vi "Recursive Add Item References to Map.vi"(8 "error in (no error)":errorcluster, 10 "ProjectItem Refnum":refnum<vi>, 11 "Icon Decorator In":refnum<class "Icon Decorator.lvclass">) -> (0 "error out":errorcluster, 3 "Icon Decorator Out":refnum<class "Icon Decorator.lvclass">)   [LabVIEW 2020, in "Icon Decorator.lvlib" / "Icon Decorator.lvclass"]
uses:
  Icon Decorator.lvclass
  Icon Decorator.lvclass/Icon Decorator.ctl
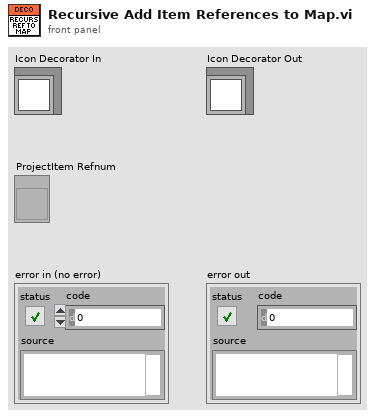
[diagram p1: front panel]
types:
  T1 = typedef "ItemRef.ctl" = u64
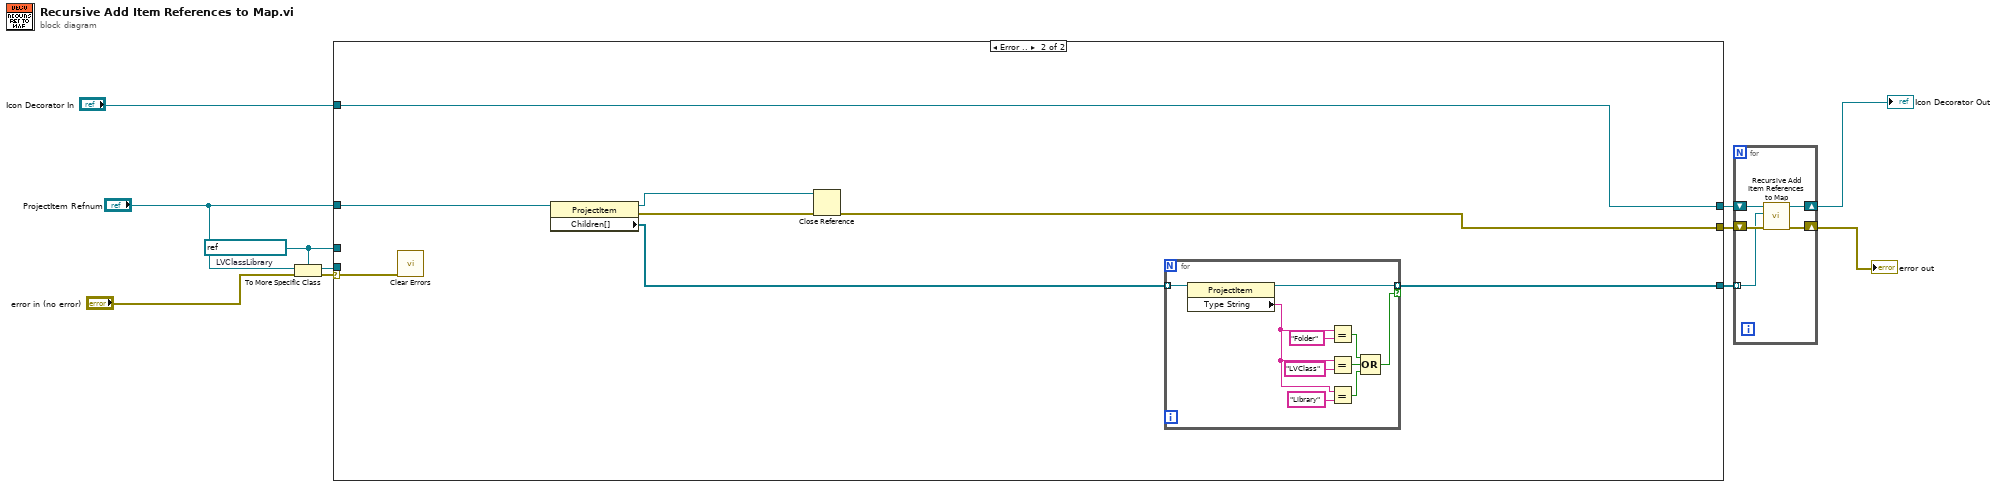
[diagram p0: block diagram]
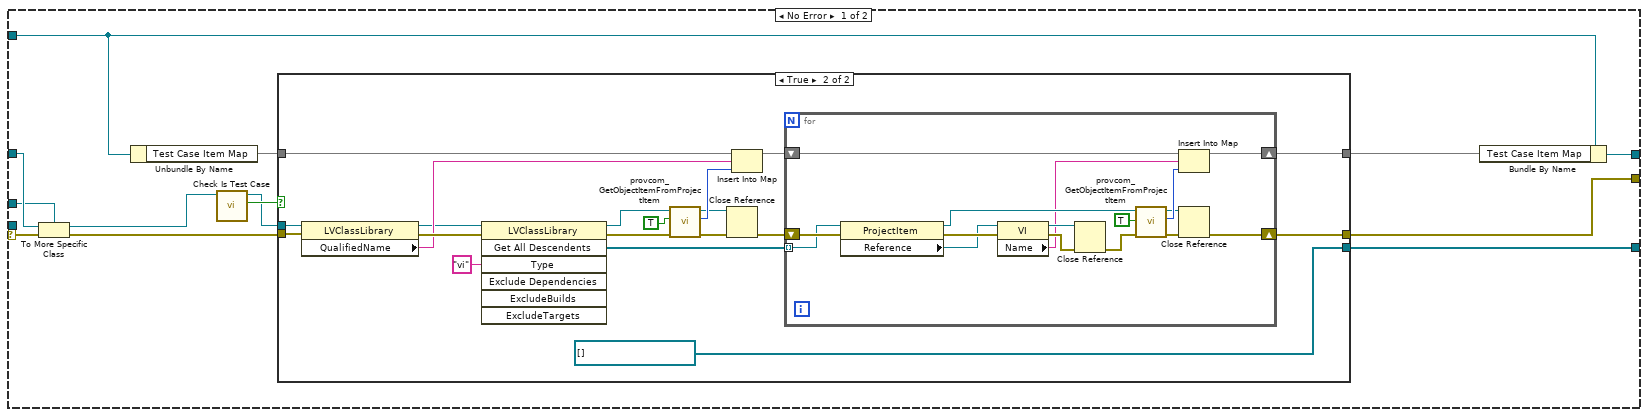
[diagram p2: hidden frame]
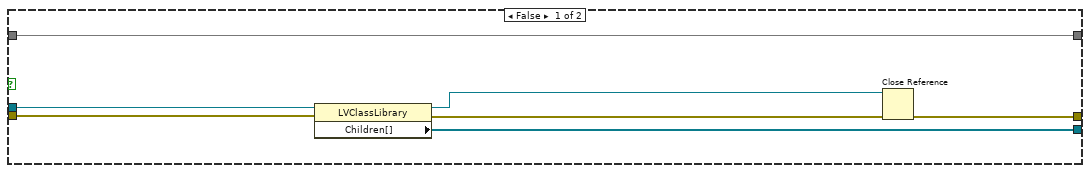
[diagram p3: hidden frame]
diagram:
  w1 = refnum<vi> refnum  # LVClassLibrary
  n1 = To More Specific Class(target class=w1, reference="ProjectItem Refnum", error in="error in (no error)") -> (specific class reference=w3:refnum<vi>, error out=w4:errorcluster)
  n2 = case shown="Error .." w4 {
    selector: w4 -> [w18 w71]
    tunnel: "Icon Decorator In" -> [w24 w69]
    tunnel: [w21 w70] -> w10
    tunnel: [w20 w69] -> w8
    tunnel: [w19 w67] -> w6
    tunnel: w3 -> [_ _]
    tunnel: "ProjectItem Refnum" -> [w16 w72]
    tunnel: w1 -> [w15 _]
    frame No Error {
      n3 = To More Specific Class(target class=w15, reference=w16, error in=w18) -> (specific class reference=w13:refnum<vi>, error out=w17:errorcluster)
      n4 = Unbundle By Name(w24) -> ("Test Case Item Map"=w22:map{string, T1})
      n5 = call "Check Is Test Case.vi"("reference in"=w13) -> ("Is Test Case?"=w14:bool, "reference out"=w12:refnum<vi>)  [unwired: 9 in]
      n6 = case shown="True" w14 {
        tunnel: w22 -> [w30 w49]
        tunnel: w12 -> [w27 w48]
        tunnel: w17 -> [w26 w43]
        tunnel: [w31 w33] -> w21
        tunnel: [w30 w35] -> w23
        tunnel: [w25 refnum<vi>[] [] ("Children[]")] -> w19
        frame False {
          n7 = property class="LVClassLibrary"(reference=w27, error in=w26) -> (reference out=w29:refnum<vi>, error out=w28:errorcluster, "Children[]"=w25:refnum<vi>[])
          n8 = Close Reference(reference=w29, error in (no error)=w28) -> (error out=w31:errorcluster)
        }
        frame True {
          n9 = property class="LVClassLibrary"(reference=w48, error in=w43) -> (reference out=w38:refnum<vi>, error out=w42:errorcluster, "QualifiedName"=w41:string)
          n10 = invoke class="LVClassLibrary" method="Get All Descendents"(reference=w38, error in=w42, "Type"="vi") -> (reference out=w37:refnum<vi>, error out=w39:errorcluster, "All Descendents"=w32:refnum<vi>[])  [unwired: 4 in, 4 out]
          n11 = call <resource>:"provcom_GetObjectItemFromProjectItem.vi"("error in (no error)"=w39, "bind? (Y)"=TRUE, "ProjectItem"=w37) -> ("error out"=w45:errorcluster, "ObjectItem"=w47:T1, "dup ProjectItem"=w46:refnum<vi>)  [unwired: 6 in]
          n12 = Close Reference(reference=w46, error in (no error)=w45) -> (error out=w34:errorcluster)
          n13 = Insert Into Map(map in=w49, key=w41, value=w47) -> (map out=w44:map{string, T1})  [unwired: 2 out]
          n14 = for {
            tunnel: w32 -> [w62] mode=indexing
            shift-right: [w65] -> w35
            shift-left: w44 -> [w66]
            shift-right: [w60] -> w33
            shift-left: w34 -> [w64]
            n15 = property class="ProjectItem"(reference=w62, error in=w64) -> (reference out=w61:refnum<vi>, error out=w63:errorcluster, "Reference"=w59:refnum<vi>)
            n16 = property class="VI"(reference=w59, error in=w63) -> (reference out=w52:refnum<vi>, error out=w54:errorcluster, "Name"=w51:string)
            n17 = Close Reference(reference=w52, error in (no error)=w54) -> (error out=w53:errorcluster)
            n18 = call <resource>:"provcom_GetObjectItemFromProjectItem.vi"("error in (no error)"=w53, "bind? (Y)"=TRUE, "ProjectItem"=w61) -> ("error out"=w57:errorcluster, "ObjectItem"=w58:T1, "dup ProjectItem"=w56:refnum<vi>)  [unwired: 6 in]
            n19 = Insert Into Map(map in=w66, key=w51, value=w58) -> (map out=w65:map{string, T1})  [unwired: 2 out]
            n20 = Close Reference(reference=w56, error in (no error)=w57) -> (error out=w60:errorcluster)
          }
        }
      }
      n21 = Bundle By Name(cluster=w24, "Test Case Item Map"=w23) -> (w20:refnum<class "Icon Decorator.lvclass">)
    }
    frame Error {
      n22 = call <vilib>:"Clear Errors.vi"("error in (no error)"=w71) -> ()  [unwired: 5 in, 2 out]
      n23 = property class="ProjectItem"(reference=w72) -> (reference out=w74:refnum<vi>, error out=w73:errorcluster, "Children[]"=w68:refnum<vi>[])  [unwired: 1 in]
      n24 = Close Reference(reference=w74, error in (no error)=w73) -> (error out=w70:errorcluster)
      n25 = for {
        tunnel: w68 -> [w84] mode=indexing
        tunnel: [w82] -> w67 mode=indexing if=w79
        n26 = property class="ProjectItem"(reference=w84) -> (reference out=w82:refnum<vi>, "Type String"=w76:string)  [unwired: 1 in, 1 out]
        n27 = Equal?(x=w76, y="Folder") -> (x = y?=w80:bool)
        n28 = Equal?(x=w76, y="LVClass") -> (x = y?=w78:bool)
        n29 = Equal?(x=w76, y="Library" ("Type")) -> (x = y?=w75:bool)
        n30 = Compound Arithmetic op=OR(w80, w78, w75) -> (w79:bool)
      }
    }
  }
  n31 = for {
    shift-right: [w88] -> w9
    shift-left: w10 -> [w89]
    shift-right: [w86] -> w7
    shift-left: w8 -> [w87]
    tunnel: w6 -> [w85] mode=indexing
    n32 = call "Recursive Add Item References to Map.vi"("error in (no error)"=w89, "ProjectItem Refnum"=w85, "Icon Decorator In"=w87) -> ("error out"=w88:errorcluster, "Icon Decorator Out"=w86:refnum<class "Icon Decorator.lvclass">)  [unwired: 7 in]
  }
  "Icon Decorator Out" <- w7
  "error out" <- w9
